vi "CalculateTotalLength.vi"(8 "error in (no error)":errorcluster, 11 "VIsData":T1[](array[typedef])) -> (0 "error out":errorcluster, 2 "Wires Length (m)":dbl, 3 "Wires Length (pix)":dbl)   [LabVIEW 2020]
uses:
  _controls/_VIWiresData.ctl
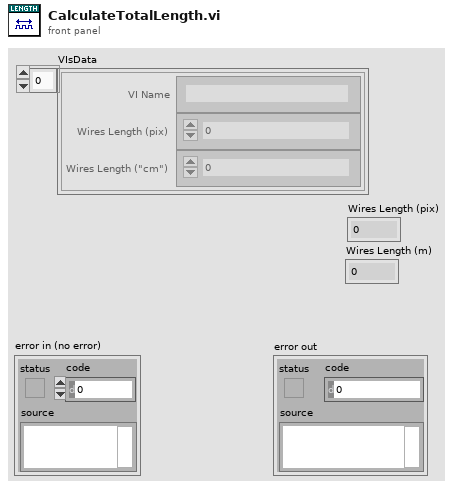
[diagram p1: front panel]
types:
  T1 = typedef "_VIWiresData.ctl" = cluster{"VI Name":string, "Wires Length (pix)":dbl, "Wires Length (\"cm\")":dbl}
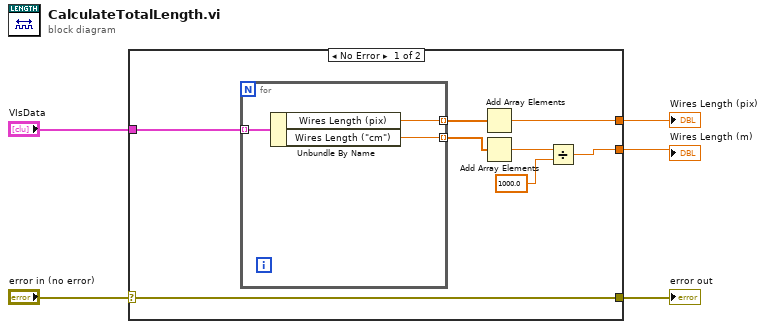
[diagram p0: block diagram]
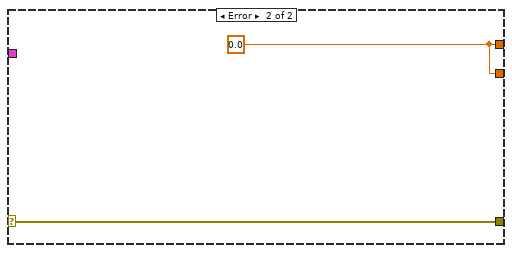
[diagram p2: hidden frame]
diagram:
  n1 = case shown="No Error" "error in (no error)" {
    selector: "error in (no error)" -> [w13 w18]
    tunnel: [w13 w18] -> w5
    tunnel: "VIsData" -> [w12 _]
    tunnel: [w9 w17] -> w2
    tunnel: [w8 w17] -> w1
    frame No Error {
      n2 = for {
        tunnel: w12 -> [w16] mode=indexing
        tunnel: [w15] -> w11 mode=indexing
        tunnel: [w14] -> w10 mode=indexing
        n3 = Unbundle By Name(w16) -> ("Wires Length (pix)"=w15:dbl, "Wires Length (\"cm\")"=w14:dbl)
      }
      n4 = Add Array Elements(numeric array=w11) -> (sum=w9:dbl)
      n5 = Add Array Elements(numeric array=w10) -> (sum=w7:dbl)
      n6 = Divide(x=w7, y=1000.0) -> (x/y=w8:dbl)
    }
    frame Error {
      w17 = 0.0 ("Wires Length (pix)")
    }
  }
  "error out" <- w5
  "Wires Length (pix)" <- w2
  "Wires Length (m)" <- w1
